vi "xxxx Core.vi"(8 "error in (no error)":errorcluster, 11 "State in":refnum<class "State.lvclass">) -> (0 "error out":errorcluster, 3 "State out":refnum<class "State.lvclass">)   [LabVIEW 2021, in "Context.lvlib" / "State.lvclass"]
uses:
  State.lvclass
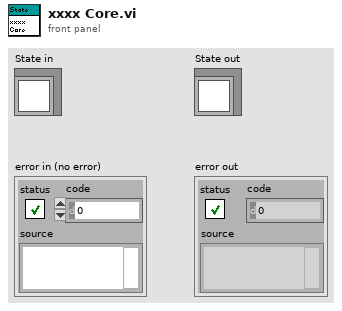
[diagram p1: front panel]
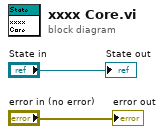
[diagram p0: block diagram]
diagram:
  "error out" <- "error in (no error)"
  "State out" <- "State in"
